vi "Sensor_Reads.vi"() -> ()   [LabVIEW 2019]
uses:
  Subsystems/Turret/Turret_Globals.vi
  Sensor_Values.vi
  <vilib>/Rock Robotics/WPI/ThirdParty/Phoenix-LabVIEW/Motor Controller/Get/CTRE_Phoenix_MotorController_GetSelectedSensorData.vi
panel:
  out "Flywheel Right":dbl
  out "Flywheel Left":dbl
  out "Turret_Spin":i32
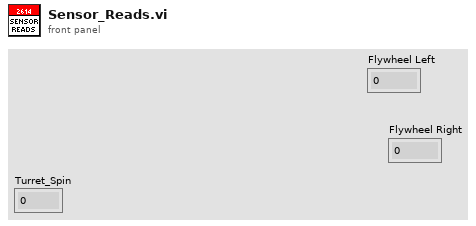
[diagram p1: front panel]
types:
  T1 = typedef "WPI_MotorControlDeviceRef.ctl" = cluster{"DeviceStatus":errorcluster, "Type":T2, "PWM":cluster{"PWM Channel":T3, "DeadBand":T4}, "CAN":cluster{"Device Number":u8, "SetOutput VI Ref":variant, "GetOutput VI Ref":variant, "Enable VI Ref":variant, "Disable VI Ref":variant, "Data":variant}, "Invert":bool, "DIO PWM":cluster{"PWM \"Enable\" Channel":T3, "DIOChannel":T5, "PWM Rate":dbl}}
  T2 = typedef "WPI_MotorControlType.ctl" = enum16{"PWM", "CAN", "DIO PWM"}
  T3 = typedef "FPGA_DIOPWMChannel.ctl" = enum8{"PWM 0", "PWM 1", "PWM 2", "PWM 3", "PWM 4", "PWM 5", "PWM 6", "PWM 7", "PWM 8", "PWM 9", "PWM MXP 0", "PWM MXP 1", "PWM MXP 2", "PWM MXP 3", "PWM MXP 4", "PWM MXP 5", "PWM MXP 6", "PWM MXP 7", "PWM MXP 8", "PWM MXP 9", "Invalid"}
  T4 = typedef "WPI_PWMDeadband.ctl" = cluster{"Name":string, "maxPositivePwm":i32, "minPositivePwm":i32, "centerPwm":i32, "maxNegativePwm":i32, "minNegativePwm":i32, "angularRange":u16}
  T5 = typedef "FPGA_DIOChannel.ctl" = enum8{"DIO 0", "DIO 1", "DIO 2", "DIO 3", "DIO 4", "DIO 5", "DIO 6", "DIO 7", "DIO 8", "DIO 9", "DIO MXP 0", "DIO MXP 1", "DIO MXP 2", "DIO MXP 3", "DIO MXP 4", "DIO MXP 5", "DIO MXP 6", "DIO MXP 7", "DIO MXP 8", "DIO MXP 9", "DIO MXP 10", "DIO MXP 11", "DIO MXP 12", "DIO MXP 13", "DIO MXP 14", "DIO MXP 15", "SPI Port CS1", "SPI Port CS2", "SPI Port CS3", "SPI Port MISO", "SPI Port MOSI", "Invalid"}
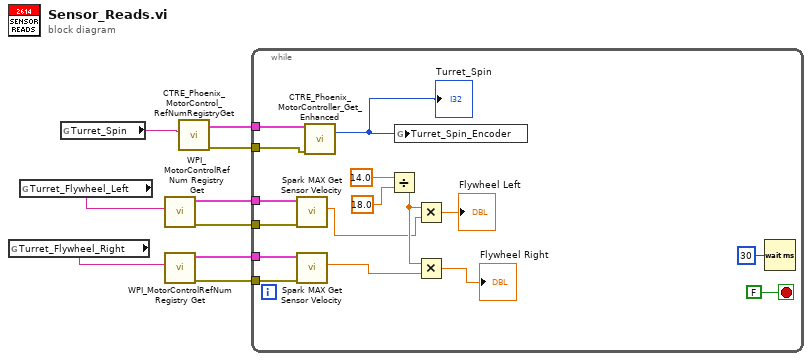
[diagram p0: block diagram]
diagram:
  n1 = global read "Turret_Globals.vi" "Turret_Flywheel_Right"() -> (w6:string)
  n2 = global read "Turret_Globals.vi" "Turret_Flywheel_Left"() -> (w5:string)
  n3 = global read "Turret_Globals.vi" "Turret_Spin"() -> (w9:string)
  n4 = call <vilib>:"WPI_MotorControlRefNum Registry Get.vi"("refnum name"=w5) -> ("error out"=w1:errorcluster, "MotorControlDevRef"=w2:T1)  [unwired: 9 in]
  n5 = call <vilib>:"WPI_MotorControlRefNum Registry Get.vi"("refnum name"=w6) -> ("error out"=w3:errorcluster, "MotorControlDevRef"=w4:T1)  [unwired: 9 in]
  n6 = call <vilib>:"CTRE_Phoenix_MotorControl_RefNumRegistryGet.vi"("refnum name"=w9) -> ("error out"=w7:errorcluster, "PhoenixMotorControlDevRef"=w8:T1)  [unwired: 9 in]
  n7 = while {
    tunnel: w8 -> [w23]
    tunnel: w7 -> [w22]
    tunnel: w4 -> [w20]
    tunnel: w3 -> [w19]
    tunnel: w2 -> [w18]
    tunnel: w1 -> [w17]
    stop <- FALSE stop-if-true
    n8 = call <vilib>:"Spark MAX Get Sensor Velocity.vi"("error in (no error)"=w17, "MotorControlDevRef in"=w18) -> ("Sensor Velocity"=w11:dbl)  [unwired: 6 in, 3 out]
    n9 = call <vilib>:"Spark MAX Get Sensor Velocity.vi"("error in (no error)"=w19, "MotorControlDevRef in"=w20) -> ("Sensor Velocity"=w10:dbl)  [unwired: 6 in, 3 out]
    n10 = call-poly <vilib>:"CTRE_Phoenix_MotorController_Get_Enhanced.vi"("PhoenixMotorControlDevRef"=w23, "error in"=w22) -> ("Position (Raw Sensor Units)"=w21:i32)  [unwired: 10 in, 3 out]
    "Turret_Spin" <- w21
    n11 = Divide(x=14.0, y=18.0) -> (x/y=w14:dbl)
    n12 = global write "Sensor_Values.vi" "Turret_Spin_Encoder"(w21) -> ()
    n13 = Multiply(x=w14, y=w11) -> (x*y=→"Flywheel Left":dbl)
    n14 = Multiply(x=w14, y=w10) -> (x*y=→"Flywheel Right":dbl)
    n15 = Wait (ms)(milliseconds to wait=u32 30) -> ()  [unwired: 1 out]
  }
